vi "7_Coincidences-JaggedArrayInLabVIEW.vi"(8 "error in (no error)":errorcluster) -> (0 "error out":errorcluster)   [LabVIEW 2014]
uses:
  SwabianInstruments.TimeTagger
panel:
  out "XY Graph":cluster{dbl[], "getData":i32[]}[](graph)
  # "The built in test signal (~ 800 to 900 kHz) is applied at different channels at different times to show how to use the class Coincidences"
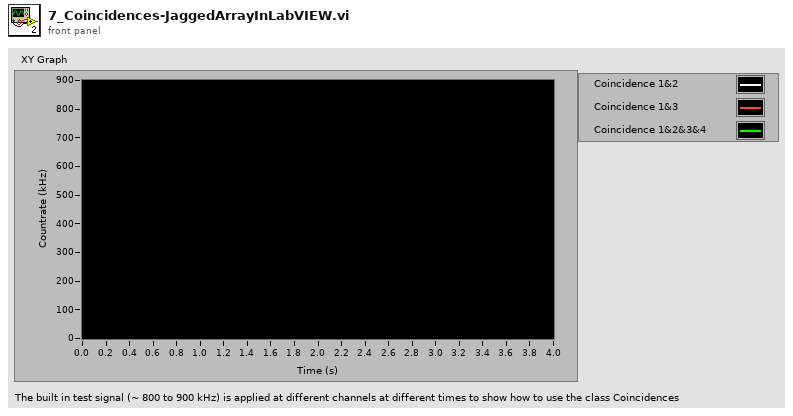
[diagram p1: front panel]
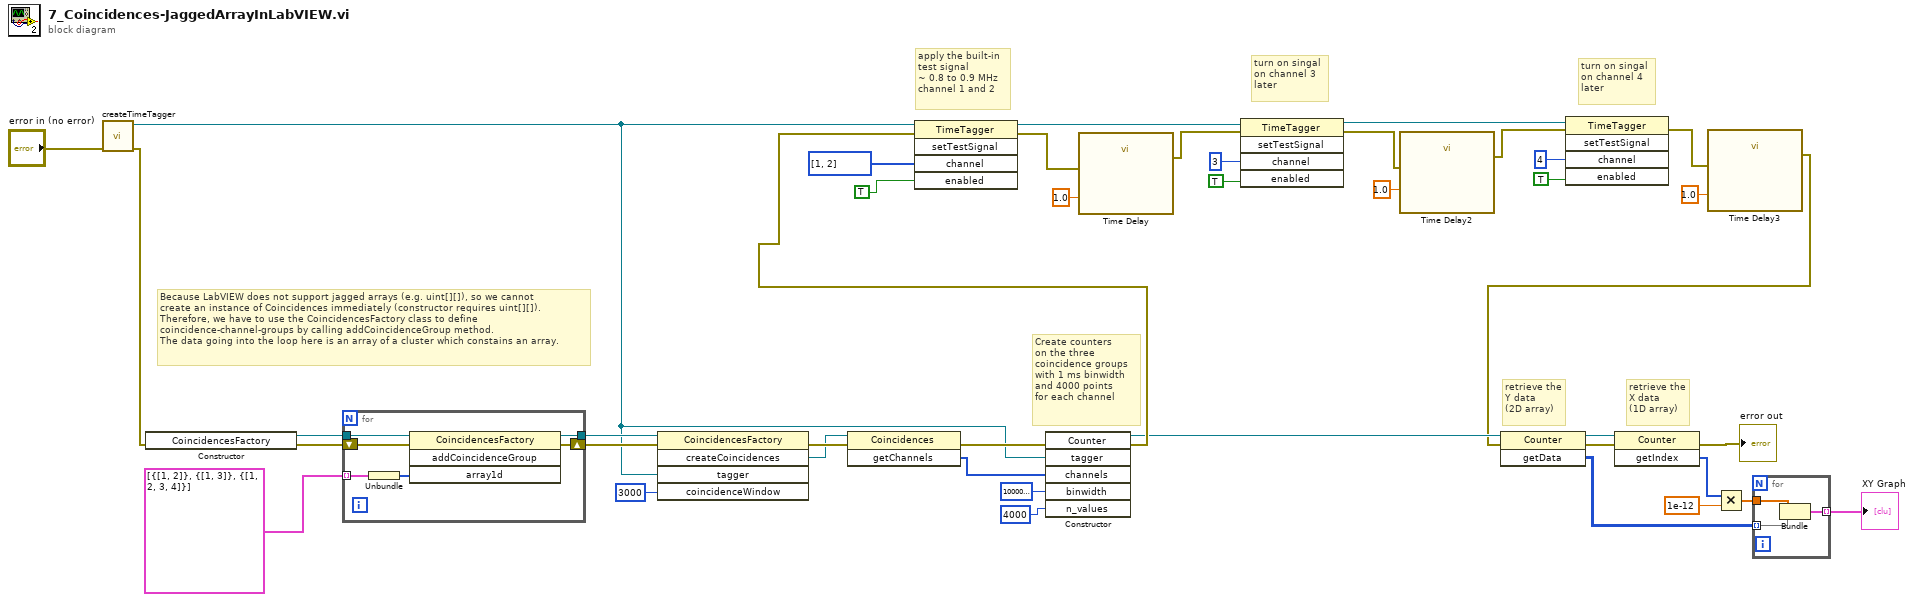
[diagram p0: block diagram]
diagram:
  # "turn on singal\non channel 4\nlater"
  # "turn on singal\non channel 3\nlater"
  # "apply the built-in\ntest signal\n~ 0.8 to 0.9 MHz\nchannel 1 and 2"
  # "Because LabVIEW does not support jagged arrays (e.g. uint[][]), so we cannot \ncreate an instance of Coincidences immediately (constructor requires uint[][]).\nTherefore, we have to use the CoincidencesFactory class to define \ncoincidence-channel-groups by calling addCoincidenceGroup method.\nThe data going into the loop here is an array of a cluster which constains an array."
  # "retrieve the\nX data\n(1D array)"
  # "retrieve the\nY data\n(2D array)"
  # "Create counters\non the three \ncoincidence groups\nwith 1 ms binwidth\nand 4000 points\nfor each channel"
  n1 = call "createTimeTagger.vi"("error in (no error)"="error in (no error)") -> ("error out"=w26:errorcluster, "TimeTagger ref out"=w25:refnum<k24>)  [unwired: 9 in]
  n2 = constructor class="CoincidencesFactory"(error in=w26) -> (reference out=w31:refnum<k24>, error out=w24:errorcluster)  [unwired: 2 in, 1 out]
  n3 = for {
    tunnel: cluster{i32[]}[] [{[1, 2]}, {[1, 3]}, {[1, 2, 3, 4]}] -> [w48] mode=indexing
    tunnel: w31 -> [w46]
    tunnel: [w45] -> w30
    shift-right: [w44] -> w29
    shift-left: w24 -> [w43]
    n4 = Unbundle(w48) -> (w47:i32[])
    n5 = invoke class="CoincidencesFactory" method="addCoincidenceGroup"(reference=w46, error in=w43, "array1d"=w47) -> (reference out=w45:refnum<k24>, error out=w44:errorcluster)  [unwired: 1 in, 2 out]
  }
  n6 = invoke class="CoincidencesFactory" method="createCoincidences"(reference=w30, error in=w29, "tagger"=w25, "coincidenceWindow"=i64 3000) -> (error out=w34:errorcluster, "createCoincidences"=w33:refnum<k24>)  [unwired: 1 in, 3 out]
  n7 = invoke class="Coincidences" method="getChannels"(reference=w33, error in=w34) -> (error out=w36:errorcluster, "getChannels"=w27:i32[])  [unwired: 1 in, 1 out]
  n8 = constructor class="Counter"(error in=w36, "tagger"=w25, "channels"=w27, "binwidth"=i64 1000000000, "n_values"=4000) -> (reference out=w39:refnum<k24>, error out=w40:errorcluster)  [unwired: 2 in, 5 out]
  n9 = invoke class="TimeTagger" method="setTestSignal"(reference=w25, error in=w40, "channel"=i32[] [1, 2], "enabled"=TRUE) -> (reference out=w1:refnum<k24>, error out=w2:errorcluster)  [unwired: 1 in, 3 out]
  n10 = call "Time Delay"("error in (no error)"=w2, "Delay Time (s)"=1.0) -> ("error out"=w12:errorcluster)  [unwired: 9 in]
  n11 = invoke class="TimeTagger" method="setTestSignal"(reference=w1, error in=w12, "channel"=3, "enabled"=TRUE) -> (reference out=w4:refnum<k24>, error out=w10:errorcluster)  [unwired: 1 in, 3 out]
  n12 = call "Time Delay2"("error in (no error)"=w10, "Delay Time (s)"=1.0) -> ("error out"=w6:errorcluster)  [unwired: 9 in]
  n13 = invoke class="TimeTagger" method="setTestSignal"(reference=w4, error in=w6, "channel"=4, "enabled"=TRUE) -> (error out=w5:errorcluster)  [unwired: 1 in, 4 out]
  n14 = call "Time Delay3"("error in (no error)"=w5, "Delay Time (s)"=1.0) -> ("error out"=w28:errorcluster)  [unwired: 9 in]
  n15 = invoke class="Counter" method="getData"(reference=w39, error in=w28) -> (reference out=w38:refnum<k24>, error out=w37:errorcluster, "getData"=w21:i32[][])  [unwired: 1 in]
  n16 = invoke class="Counter" method="getIndex"(reference=w38, error in=w37) -> (error out=→"error out":errorcluster, "getIndex"=w20:i64[])  [unwired: 1 in, 1 out]
  n17 = Multiply(x=w20, y=1e-12) -> (x*y=w22:dbl[])
  n18 = for {
    tunnel: w21 -> [w50] mode=indexing
    tunnel: w22 -> [w51]
    tunnel: [w49] -> w19 mode=indexing
    n19 = Bundle(w51, "getData"=w50) -> (w49:cluster{dbl[], "getData":i32[]})  [unwired: 1 in]
  }
  "XY Graph" <- w19
